vi "getFrequency.vi"(0 "BK1823ACounter.lvclass":refnum<class "BK1823ACounter.lvclass">, 1 "error in (no error)":errorcluster) -> (2 "BK1823ACounter.lvclass 2":refnum<class "BK1823ACounter.lvclass">, 3 "Frequency":string, 4 "error out":errorcluster)   [LabVIEW 2011, in "Hardware.lvlib" / "frequencyCounters.lvlib" / "BK1823ACounter.lvclass"]
uses:
  BK1823ACounter.lvclass
  FrequencyCounter/FrequencyCounter.lvclass
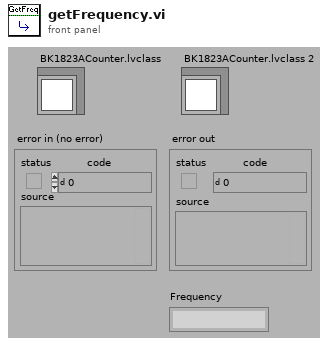
[diagram p1: front panel]
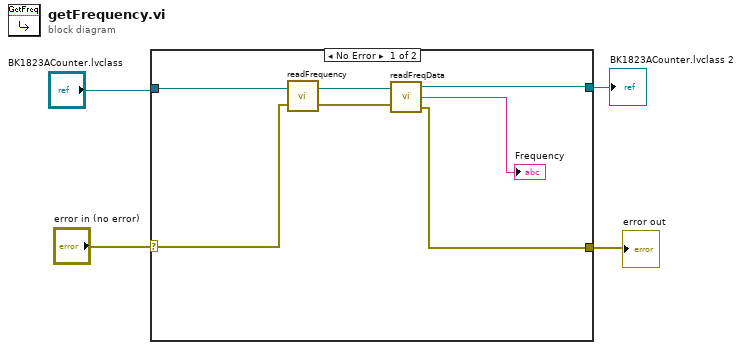
[diagram p0: block diagram]
diagram:
  n1 = case shown="No Error" "error in (no error)" {
    selector: "error in (no error)" -> [w10 w12]
    tunnel: "BK1823ACounter.lvclass" -> [w11 w13]
    tunnel: [w7 w13] -> w2
    tunnel: [w6 w12] -> w1
    frame No Error {
      n2 = call "readFrequency.vi"("error in (no error)"=w10, "BK1823ACounter.lvclass"=w11) -> ("error out"=w8:errorcluster, "BK1823ACounter.lvclass 2"=w9:refnum<class "BK1823ACounter.lvclass">)
      n3 = call "readFreqData.vi"("FrequencyCounter.lvclass"=w9, "error in (no error)"=w8) -> ("FrequencyCounter.lvclass 2"=w7:refnum<class "BK1823ACounter.lvclass">, "String"=→"Frequency":string, "error out"=w6:errorcluster)
    }
    frame Error {
    }
  }
  "error out" <- w1
  "BK1823ACounter.lvclass 2" <- w2
